vi "Bookmarks.vi"(8 "Error In":errorcluster, 10 "VIs":T1[](array[typedef]), 11 "Project Target App In":refnum<vi>) -> (0 "Error Out":errorcluster, 2 "Bookmarks":T3, 3 "Project Target App Out":refnum<vi>)   [LabVIEW 2017, in "Graveyard.lvlib"]
uses:
  Graveyard.lvlib
  <vilib>/Utility/miscctls.llb/LVBookmarkInfoTypeDef.ctl
  VI Information.ctl
  Application Information.ctl
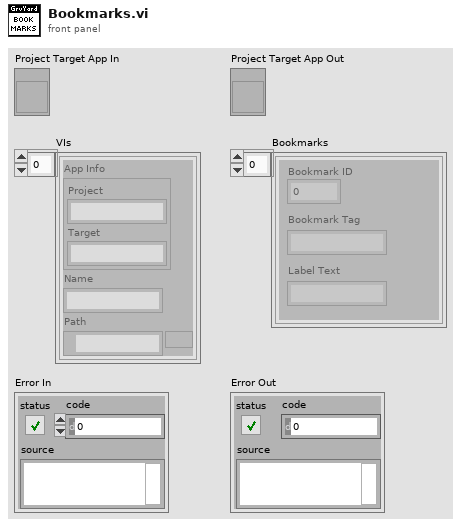
[diagram p1: front panel]
types:
  T1 = typedef "Graveyard.lvlib/VI Information.ctl" = cluster{"App Info":T2, "Name":string, "Path":path}
  T2 = typedef "Graveyard.lvlib/Application Information.ctl" = cluster{"Project":string, "Target":string}
  T3 = typedef "LVBookmarkInfoTypeDef.ctl" = cluster{"Bookmark ID":u32, "Bookmark Tag":string, "Label Text":string}[]
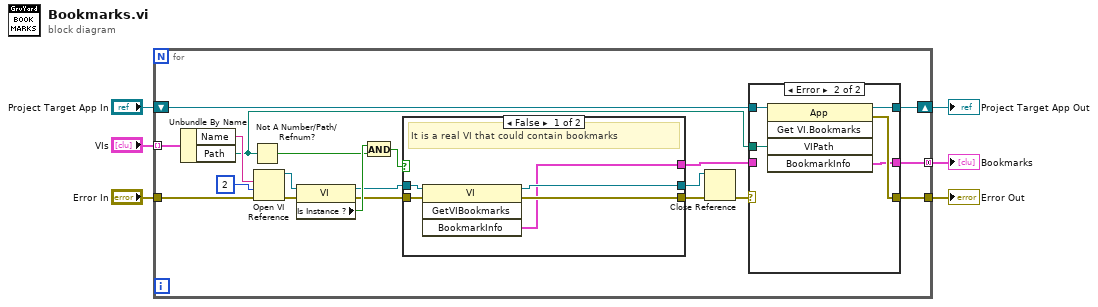
[diagram p0: block diagram]
diagram:
  n1 = for {
    tunnel: "Error In" -> [w26]
    tunnel: "VIs" -> [w24] mode=indexing
    shift-right: [w9] -> w5
    shift-left: "Project Target App In" -> [w10]
    tunnel: [w8] -> w4
    tunnel: [w7] -> w6 mode=concatenating
    n2 = Unbundle By Name(w24) -> ("Name"=w12:string, "Path"=w11:path)
    n3 = Not A Number/Path/Refnum?(number/path/refnum=w11) -> (NaN/Path/Refnum?=w20:bool)
    n4 = Open VI Reference(vi path=w12, options=2, error in (no error)=w26) -> (vi reference=w22:refnum<vi>, error out=w23:errorcluster)  [unwired: 3 in]
    n5 = property class="VI"(reference=w22, error in=w23) -> (reference out=w17:refnum<vi>, error out=w18:errorcluster, "Is Instance ?"=w21:bool)
    n6 = And(x=w21, y=w20) -> (x .and. y?=w19:bool)
    n7 = case shown="False" w19 {
      tunnel: w18 -> [w38 w40]
      tunnel: w17 -> [w39 w41]
      tunnel: [w37 w41] -> w16
      tunnel: [w36 w40] -> w15
      tunnel: [w35 _] -> w13
      frame False {
        # "It is a real VI that could contain bookmarks"
        n8 = invoke class="VI" method="GetVIBookmarks"(reference=w39, error in=w38) -> (reference out=w37:refnum<vi>, error out=w36:errorcluster, "BookmarkInfo"=w35:T3)  [unwired: 2 in, 1 out]
      }
      frame True {
        # "It is an Express VI or the path does not exist"
      }
    }
    n9 = Close Reference(reference=w16, error in (no error)=w15) -> (error out=w14:errorcluster)
    n10 = case shown="Error" w14 {
      selector: w14 -> [w28 _]
      tunnel: w13 -> [w29 _]
      tunnel: [w29 w33] -> w7
      tunnel: [w28 w34] -> w8
      tunnel: w11 -> [_ w32]
      tunnel: w10 -> [w27 w31]
      tunnel: [w27 w30] -> w9
      frame No Error {
      }
      frame Error {
        n11 = invoke class="App" method="Get VI.Bookmarks"(reference=w31, "VIPath"=w32) -> (reference out=w30:refnum<vi>, error out=w34:errorcluster, "BookmarkInfo"=w33:T3)  [unwired: 3 in, 2 out]
      }
    }
  }
  "Bookmarks" <- w6
  "Project Target App Out" <- w5
  "Error Out" <- w4
